vi "logUpdater.vi"(1 "Response":refnum<vi>, 2 "Input":string) -> (0 "concatenated string":string)   [LabVIEW 2015]
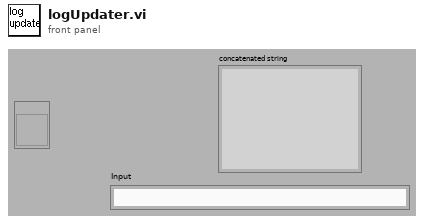
[diagram p1: front panel]
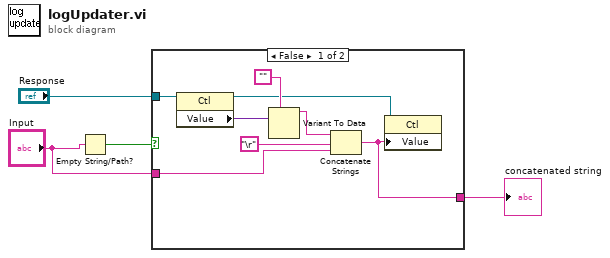
[diagram p0: block diagram]
diagram:
  n1 = Empty String/Path?(string/path="Input") -> (empty?=w1:bool)
  n2 = case shown="False" w1 {
    tunnel: "Response" -> [w12 _]
    tunnel: [w7 _] -> w3
    tunnel: "Input" -> [w5 _]
    frame False {
      n3 = property class="Ctl"(reference=w12) -> (reference out=w9:refnum<vi>, "Value"=w11:variant)  [unwired: 1 in, 1 out]
      n4 = Variant To Data(type="", Variant=w11) -> (data=w8:string)  [unwired: 1 in, 1 out]
      n5 = Concatenate Strings(w8, "\r", w5) -> (w7:string)
      n6 = property class="Ctl"(reference=w9, "Value"=w7) -> ()  [unwired: 1 in, 2 out]
    }
    frame True {
    }
  }
  "concatenated string" <- w3
